vi "HRTF-Sort Filestems.vi"(7 "Filestems":string[](array[string])) -> (8 "Sorted filestems":string[](array[string]))   [LabVIEW 2015]
uses:
  <vilib>/regexp/Match Regular Expression.xnode
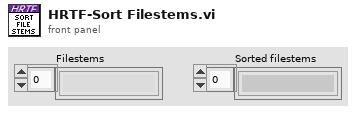
[diagram p1: front panel]
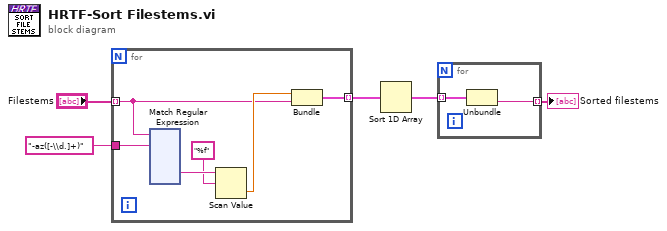
[diagram p0: block diagram]
diagram:
  n1 = for {
    tunnel: "-az([-\\d.]+)" ("regular expression") -> [w11]
    tunnel: "Filestems" -> [w7] mode=indexing
    tunnel: [w6] -> w3 mode=indexing
    n2 = xnode "Match Regular Expression"("input string"=w7, "regular expression"=w11) -> ("submatch 1"=w10:string)  [unwired: 4 in, 6 out]
    n3 = Scan Value(string=w10, format string="%f") -> (value=w8:dbl)  [unwired: 1 in, 1 out]
    n4 = Bundle(w8, w7) -> (w6:cluster{dbl, string})  [unwired: 1 in]
  }
  n5 = Sort 1D Array(array=w3) -> (sorted array=w2:cluster{dbl, string}[])
  n6 = for {
    tunnel: w2 -> [w130] mode=indexing
    tunnel: [w129] -> w1 mode=indexing
    n7 = Unbundle(w130) -> (w129:string)  [unwired: 1 out]
  }
  "Sorted filestems" <- w1
